vi "lighting control1.vi"() -> ()   [LabVIEW 2021]
uses:
  <vilib>/MakerHub/LINX/Public/Peripherals/Digital/Digital Write N Chans.vi
  9d78b206-77b7-4c78-aba5-ec40e68928b8.vi
  9e639ab3-c25c-4c4a-bd12-325d10f84e49.vi
  <vilib>/MakerHub/LINX/Private/Local IO/LinxDigitalWrite.vi
  <vilib>/MakerHub/LINX/Public/Utilities/Check Channel.vi
  <vilib>/MakerHub/LINX/Private/Local IO/LinxI2cWrite.vi
  <vilib>/MakerHub/LINX/Public/Utilities/Open Serial.vi
  <vilib>/Utility/file.llb/Write Delimited Spreadsheet (string).vi
  <vilib>/MakerHub/LINX/Private/Utilties/Generate Error.vi
  <vilib>/addons/Fuzzy Logic/FL Fuzzy Controller (MISO).vi
  <vilib>/Utility/file.llb/Write Delimited Spreadsheet (DBL).vi
  <vilib>/MakerHub/LINX/LMH-LINX.lvlib
  <vilib>/addons/Fuzzy Logic/NI_Fuzzy_Logic_API.lvlib
panel:
  out "no lamps":dbl
  out "fuzzy output":dbl
  out "no lamps":dbl
  out "fuzzy output":dbl
  out "indoor real":dbl
  in  "?":bool[](array[boolean])
  in  "?":bool[](array[boolean])
  in  "?":bool[](array[boolean])
  in  "Relay channels 3":dbl[](array[numeric])
  in  "outer stop":bool
  in  "inner stop":bool
  in  "channel name":string[](array[string])
  in  "Relay channels 2":dbl[](array[numeric])
  in  "Array 16":bool[](array[boolean])
  in  "Array 15":bool[](array[boolean])
  in  "?":bool[](array[boolean])
  in  "?":bool[](array[boolean])
  in  "?":bool[](array[boolean])
  in  "?":bool[](array[boolean])
  in  "?":bool[](array[boolean])
  in  "?":bool[](array[boolean])
  out "indoor from regr":dbl
  out "outdoor 2":dbl
  in  "Array 8":bool[](array[boolean])
  in  "Array 7":bool[](array[boolean])
  in  "?":bool[](array[boolean])
  in  "?":bool[](array[boolean])
  in  "?":bool[](array[boolean])
  in  "?":bool[](array[boolean])
  in  "?":bool[](array[boolean])
  in  "?":bool[](array[boolean])
  in  "Relay channels":dbl[](array[numeric])
  out "outdoor":dbl
  out "indoor":dbl
  # "CSV COLUMN CONFIG"
  # "RELAY ARDUINO CHANNELS"
  # "OFF CONFIG"
  # "DATA"
  # "BULB CASE CONFIG"
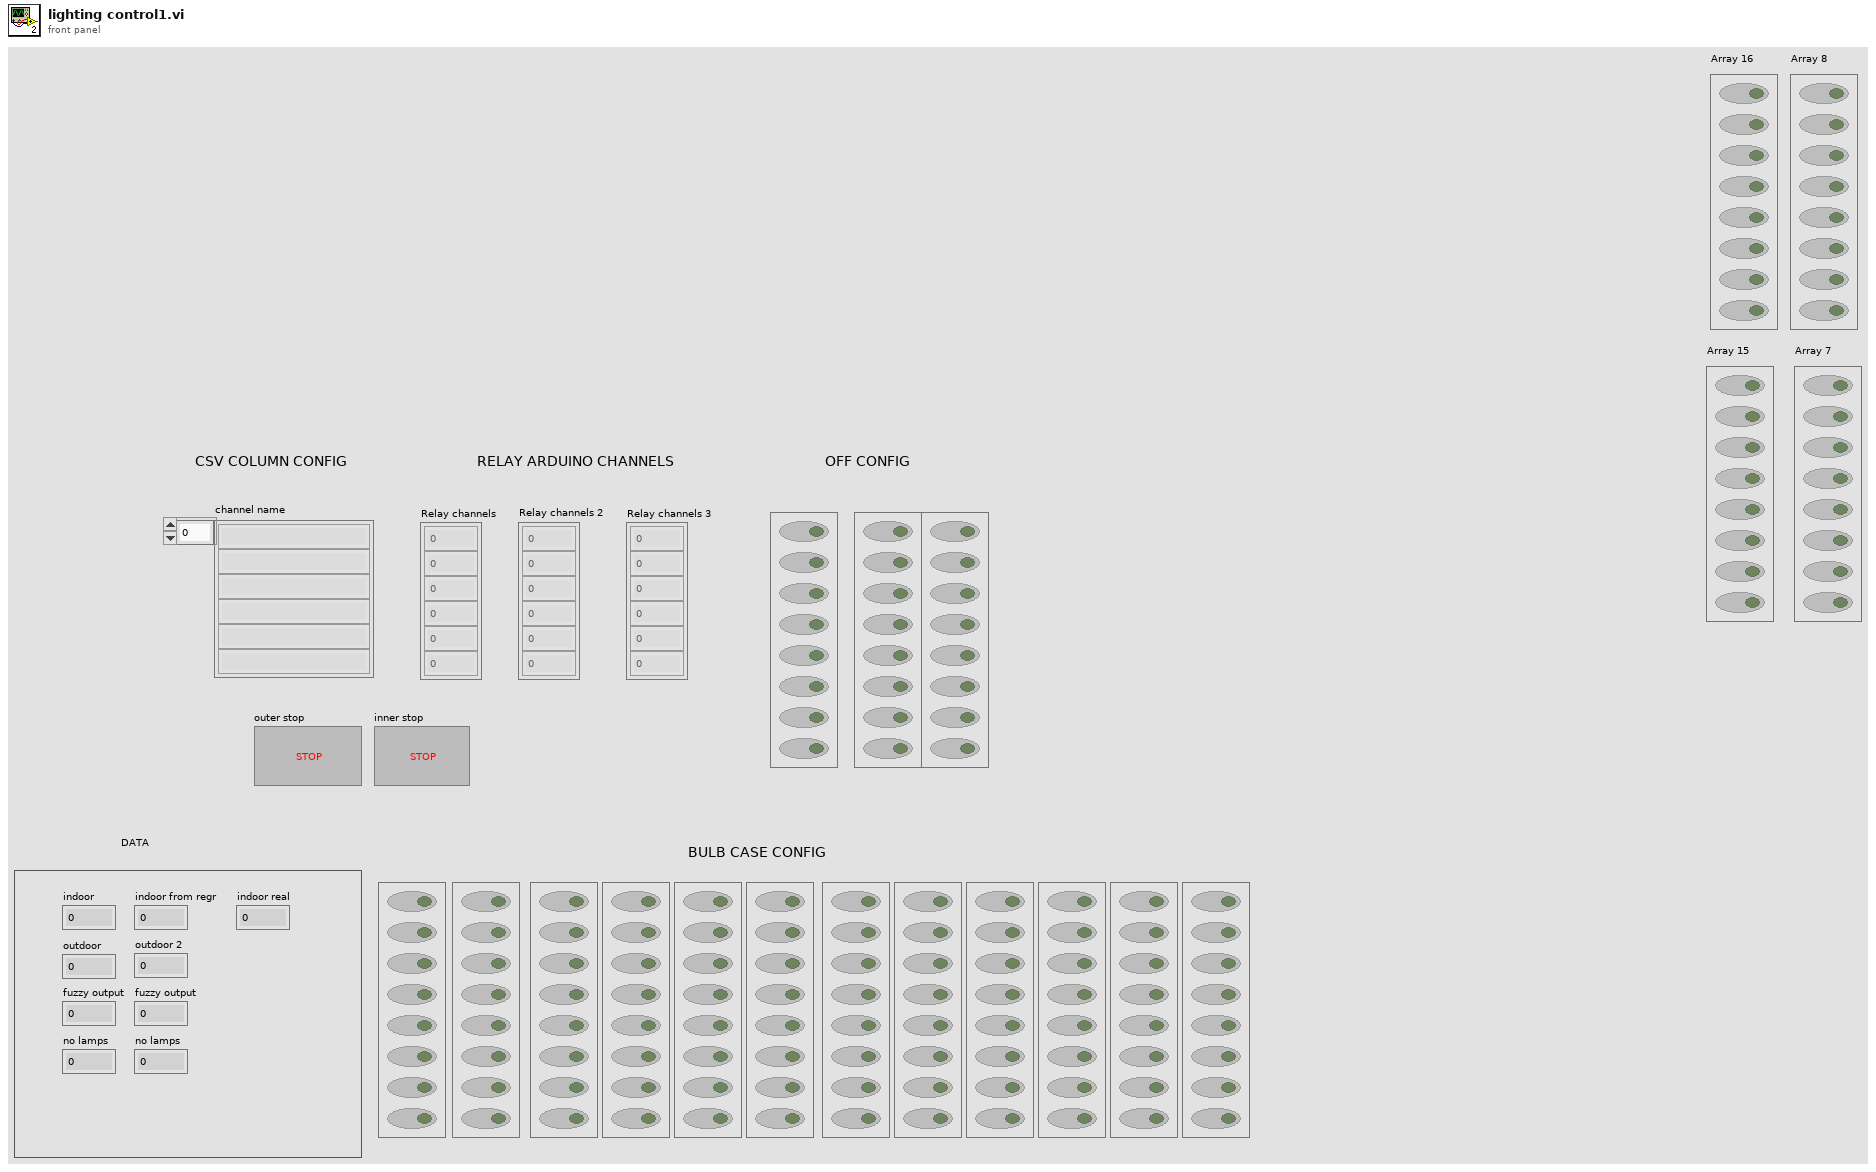
[diagram p1: front panel]
types:
  T1 = typedef "LMH-LINX.lvlib/LINX Ref.ctl" = cluster{"IO":T2, "Interface":T3, "LINX Device Config":T4}
  T2 = typedef "LMH-LINX.lvlib/Platform.ctl" = enum16{"Remote", "Local"}
  T3 = typedef "LMH-LINX.lvlib/Interface.ctl" = enum16{"Serial", "TCP"}
  T4 = typedef "LMH-LINX.lvlib/Device.lvlib/LINX Device Config.ctl" = cluster{"Interface":T3, "COM Port":refnum<visa-resource-name>, "TCP Configuration":T5, "Device Family":u8, "Device ID":u8, "Device Name":string, "TCP Ref":refnum<k5>, "Channels":T6}
  T5 = typedef "LMH-LINX.lvlib/Device.lvlib/TCP Config.ctl" = cluster{"IP Address":string, "Port":u16}
  T6 = typedef "LMH-LINX.lvlib/Channels.ctl" = cluster{"DI":u8[], "DO":u8[], "AI":u8[], "AO":u8[], "PWM":u8[], "QE":u8[], "UART":u8[], "I2C 2":u8[], "SPI":u8[], "CAN":u8[], "Servo":u8[], "AI Ref (V)":dbl, "AI Resolution (Bits)":u8, "AO Ref (V)":dbl, "AO Resolution (Bits)":u8}
  T7 = typedef "NI_Fuzzy_Logic_API.lvlib/FL System.ctl" = cluster{"input variables":T8[], "output variables":T8[], "rules":T11[], "defuzzification method":T17, "description":string, "user MF interpolating polynomials":T18[]}
  T8 = typedef "NI_Fuzzy_Logic_API.lvlib/FL Variable.ctl" = cluster{"name":string, "range":dbl[], "MFs":T9[]}
  T9 = typedef "NI_Fuzzy_Logic_API.lvlib/FL Membership Function.ctl" = cluster{"name":string, "shape":T10, "points":dbl[], "color":u32, "user-defined shape index":i32}
  T10 = typedef "NI_Fuzzy_Logic_API.lvlib/FL Membership Function Shape.ctl" = u16
  T11 = typedef "NI_Fuzzy_Logic_API.lvlib/FL Rule.ctl" = cluster{"antecedents":T12[], "antecedent connective":T14, "consequents":T15[], "consequent implication":T16, "degree of support":dbl}
  T12 = typedef "NI_Fuzzy_Logic_API.lvlib/FL Antecedent.ctl" = cluster{"Var Index":i32, "MF Index":i32, "Cond":T13}
  T13 = typedef "NI_Fuzzy_Logic_API.lvlib/FL Modifier.ctl" = u16
  T14 = typedef "NI_Fuzzy_Logic_API.lvlib/FL Antecedent Connective.ctl" = u16
  T15 = typedef "NI_Fuzzy_Logic_API.lvlib/FL Consequent.ctl" = cluster{"Var Index":i32, "MF Index":i32, "Cond":T13}
  T16 = typedef "NI_Fuzzy_Logic_API.lvlib/FL Consequent Implication.ctl" = u16
  T17 = typedef "NI_Fuzzy_Logic_API.lvlib/FL Defuzzification.ctl" = u16
  T18 = typedef "NI_Fuzzy_Logic_API.lvlib/FL Interpolating polynomials.ctl" = cluster{"X":dbl[], "Y":dbl[], "Y(x) coeff":dbl[][], "X(y) coeff":dbl[][], "Area(y) coeff":dbl[][], "coa_x(y) coeff":dbl[][]}
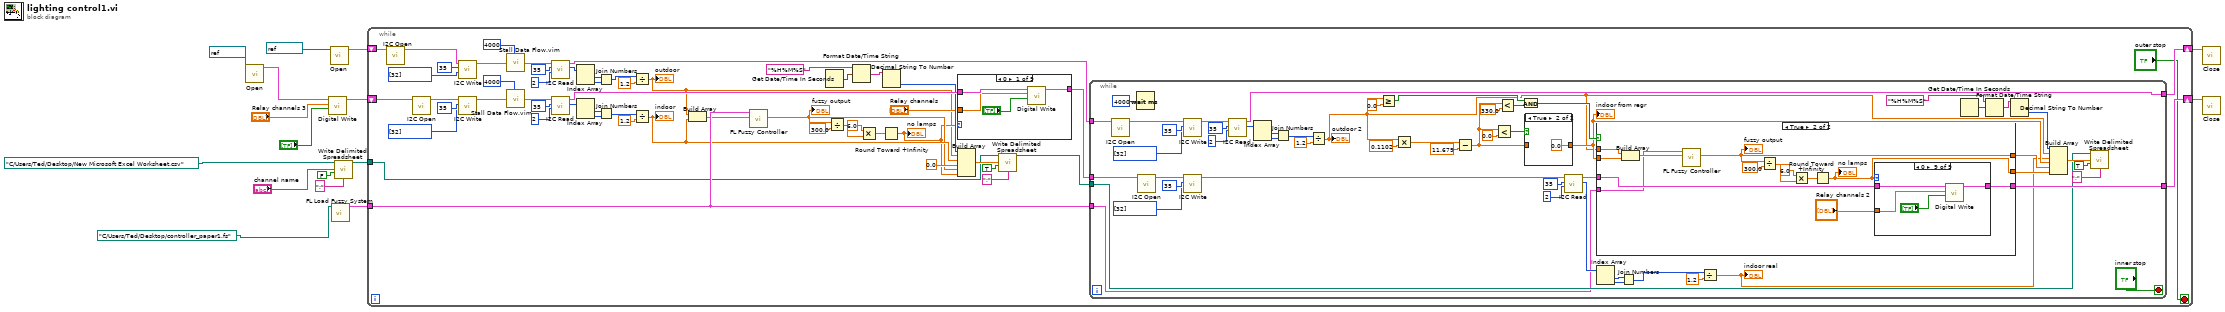
[diagram p0: block diagram]
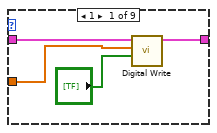
[diagram p4: hidden frame]
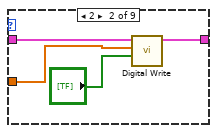
[diagram p5: hidden frame]
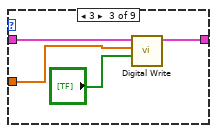
[diagram p6: hidden frame]
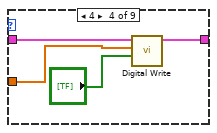
[diagram p7: hidden frame]
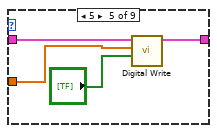
[diagram p8: hidden frame]
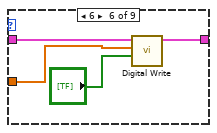
[diagram p9: hidden frame]
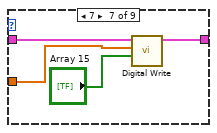
[diagram p10: hidden frame]
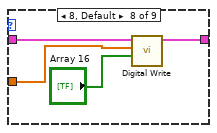
[diagram p11: hidden frame]
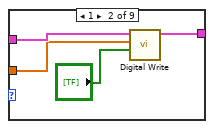
[diagram p12: hidden frame]
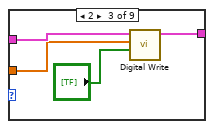
[diagram p13: hidden frame]
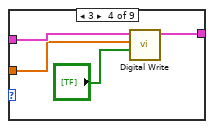
[diagram p14: hidden frame]
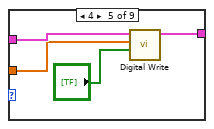
[diagram p15: hidden frame]
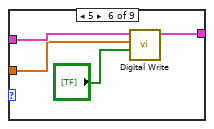
[diagram p16: hidden frame]
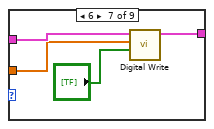
[diagram p17: hidden frame]
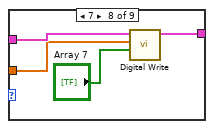
[diagram p18: hidden frame]
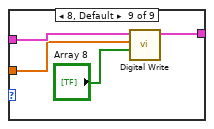
[diagram p19: hidden frame]
diagram:
  n1 = call-poly <vilib>:"Open.vi"("Serial Port"=refnum<visa-resource-name> "COM4") -> ("LINX Resource"=w2:T1)  [unwired: 8 in, 2 out]
  n2 = call-poly <vilib>:"Digital Write.vi"("Values"="?", "DO Channels"="Relay channels 3", "LINX Resource"=w2) -> ("LINX Resource"=w1:T1)  [unwired: 7 in, 1 out]
  n3 = call-poly <vilib>:"Open.vi"("Serial Port"=refnum<visa-resource-name> "COM5") -> ("LINX Resource"=w16:T1)  [unwired: 8 in, 2 out]
  n4 = call <vilib>:"FL Load Fuzzy System.vi"("file path"=path "C:/Users/Ted/Desktop/controller_paper1.fs") -> ("fuzzy system out"=w5:T7)  [unwired: 9 in, 1 out]
  n5 = call-poly <vilib>:"Write Delimited Spreadsheet.vi"("file path (dialog if empty)"=path "C:/Users/Ted/Desktop/New Microsoft Excel Worksheet.csv", "1D data"="channel name", "append to file? (new file:F)"=FALSE, "delimiter (\\t)"=";" ("delimiter (\\t)")) -> ("new file path (Not A Path if cancelled)"=w6:path)  [unwired: 10 in, 1 out]
  n6 = while {
    tunnel: w6 -> [w18]
    tunnel: w5 -> [w46]
    shift-right: [w48] -> w12
    shift-left: w1 -> [w61]
    shift-right: [w47] -> w11
    shift-left: w16 -> [w51]
    stop <- "outer stop" stop-if-true
    n7 = call <vilib>:"I2C Open.vi"("LINX Resource"=w51) -> ("LINX Resource"=w60:T1)  [unwired: 9 in, 1 out]
    n8 = call <vilib>:"I2C Open.vi"("LINX Resource"=w61) -> ("LINX Resource"=w71:T1)  [unwired: 9 in, 1 out]
    n9 = call <vilib>:"I2C Write.vi"("Data"=u8[] [32], "I2C Slave Address (0)"=u8 35, "LINX Resource"=w60) -> ("LINX Resource"=w41:T1)  [unwired: 7 in, 1 out]
    n10 = call <vilib>:"I2C Write.vi"("Data"=u8[] [32], "I2C Slave Address (0)"=u8 35, "LINX Resource"=w71) -> ("LINX Resource"=w44:T1)  [unwired: 7 in, 1 out]
    n11 = call "Stall Data Flow.vim"("value in"=w41, "milliseconds to wait"=u32 4000) -> ("value out"=w40:T1)  [unwired: 1 out]
    n12 = call "Stall Data Flow.vim"("value in"=w44, "milliseconds to wait"=u32 4000) -> ("value out"=w43:T1)  [unwired: 1 out]
    n13 = call <vilib>:"I2C Read.vi"("Bytes To Read"=u8 2, "I2C Slave Address (0)"=u8 35, "LINX Resource"=w40) -> ("Data"=w50:u8[], "LINX Resource"=w49:T1)  [unwired: 6 in, 1 out]
    n14 = call <vilib>:"I2C Read.vi"("Bytes To Read"=u8 2, "I2C Slave Address (0)"=u8 35, "LINX Resource"=w43) -> ("Data"=w68:u8[], "LINX Resource"=w45:T1)  [unwired: 6 in, 1 out]
    n15 = Index Array(array=w50) -> (element #1=w57:u8, element #2=w56:u8)  [unwired: 2 in]
    n16 = Index Array(array=w68) -> (element #1=w67:u8, element #2=w66:u8)  [unwired: 2 in]
    n17 = Join Numbers(hi=w57, lo=w56) -> ((hi.lo)=w54:u16)
    n18 = Join Numbers(hi=w67, lo=w66) -> ((hi.lo)=w64:u16)
    n19 = Divide(x=w54, y=1.2) -> (x/y=w17:dbl)
    "outdoor" <- w17
    n20 = Divide(x=w64, y=1.2) -> (x/y=w37:dbl)
    "indoor" <- w37
    n21 = Build Array(w17, w37) -> (w36:dbl[])
    n22 = call-poly <vilib>:"FL Fuzzy Controller.vi"("input values"=w36, "fuzzy system in"=w46) -> ("output value"=w20:dbl)  [unwired: 5 in, 4 out]
    "fuzzy output" <- w20
    n23 = Get Date/Time In Seconds() -> (seconds since 1Jan1904=w31:timestamp)
    n24 = Divide(x=w20, y=300.0) -> (x/y=w34:dbl)
    n25 = Format Date/Time String(time format string (%c)="%H%M%S", seconds (now)=w31) -> (date/time string=w29:string)  [unwired: 1 in]
    n26 = Multiply(x=6.0, y=w34) -> (x*y=w23:dbl)
    n27 = Decimal String To Number(string=w29) -> (number=w28:i32)  [unwired: 2 in, 1 out]
    n28 = Round Toward +Infinity(x=w23) -> (ceil(x): smallest int >= x=w19:dbl)
    "no lamps" <- w19
    n29 = case shown="0" w19 {
      tunnel: w45 -> [w181 w185 w188 w193 w196 w200 w205 w209 w213]
      tunnel: [w180 w184 w189 w192 w197 w201 w204 w208 w212] -> w32
      tunnel: "Relay channels" -> [w179 w182 w187 w191 w195 w199 w202 w207 w210]
      frame 0 {
        n30 = call-poly <vilib>:"Digital Write.vi"("Values"="?", "DO Channels"=w179, "LINX Resource"=w181) -> ("LINX Resource"=w180:T1)  [unwired: 7 in, 1 out]
      }
      frame 1 {
        n31 = call-poly <vilib>:"Digital Write.vi"("Values"="?", "DO Channels"=w182, "LINX Resource"=w185) -> ("LINX Resource"=w184:T1)  [unwired: 7 in, 1 out]
      }
      frame 2 {
        n32 = call-poly <vilib>:"Digital Write.vi"("Values"="?", "DO Channels"=w187, "LINX Resource"=w188) -> ("LINX Resource"=w189:T1)  [unwired: 7 in, 1 out]
      }
      frame 3 {
        n33 = call-poly <vilib>:"Digital Write.vi"("Values"="?", "DO Channels"=w191, "LINX Resource"=w193) -> ("LINX Resource"=w192:T1)  [unwired: 7 in, 1 out]
      }
      frame 4 {
        n34 = call-poly <vilib>:"Digital Write.vi"("Values"="?", "DO Channels"=w195, "LINX Resource"=w196) -> ("LINX Resource"=w197:T1)  [unwired: 7 in, 1 out]
      }
      frame 5 {
        n35 = call-poly <vilib>:"Digital Write.vi"("Values"="?", "DO Channels"=w199, "LINX Resource"=w200) -> ("LINX Resource"=w201:T1)  [unwired: 7 in, 1 out]
      }
      frame 6 {
        n36 = call-poly <vilib>:"Digital Write.vi"("Values"="?", "DO Channels"=w202, "LINX Resource"=w205) -> ("LINX Resource"=w204:T1)  [unwired: 7 in, 1 out]
      }
      frame 7 {
        n37 = call-poly <vilib>:"Digital Write.vi"("Values"="Array 7", "DO Channels"=w207, "LINX Resource"=w209) -> ("LINX Resource"=w208:T1)  [unwired: 7 in, 1 out]
      }
      frame 8, Default {
        n38 = call-poly <vilib>:"Digital Write.vi"("Values"="Array 8", "DO Channels"=w210, "LINX Resource"=w213) -> ("LINX Resource"=w212:T1)  [unwired: 7 in, 1 out]
      }
    }
    n39 = Build Array(w28, w17, w37, 0.0 ("element"), w20, w19) -> (w27:dbl[])
    n40 = call-poly <vilib>:"Write Delimited Spreadsheet.vi"("file path (dialog if empty)"=w18, "1D data"=w27, "append to file? (new file:F)"=TRUE, "delimiter (\\t)"=";" ("delimiter (\\t)")) -> ("new file path (Not A Path if cancelled)"=w25:path)  [unwired: 10 in, 1 out]
    n41 = while {
      tunnel: w32 -> [w103]
      tunnel: w49 -> [w102]
      tunnel: [w101] -> w48
      tunnel: [w100] -> w47
      tunnel: w25 -> [w93]
      tunnel: w46 -> [w90]
      stop <- "inner stop" stop-if-true
      n42 = call <vilib>:"I2C Open.vi"("LINX Resource"=w102) -> ("LINX Resource"=w125:T1)  [unwired: 9 in, 1 out]
      n43 = Wait (ms)(milliseconds to wait=u32 4000) -> ()  [unwired: 1 out]
      n44 = call <vilib>:"I2C Open.vi"("LINX Resource"=w103) -> ("LINX Resource"=w115:T1)  [unwired: 9 in, 1 out]
      n45 = call <vilib>:"I2C Write.vi"("Data"=u8[] [32], "I2C Slave Address (0)"=u8 35, "LINX Resource"=w125) -> ("LINX Resource"=w89:T1)  [unwired: 7 in, 1 out]
      n46 = call <vilib>:"I2C Write.vi"("Data"=u8[] [32], "I2C Slave Address (0)"=u8 35, "LINX Resource"=w115) -> ("LINX Resource"=w107:T1)  [unwired: 7 in, 1 out]
      n47 = call <vilib>:"I2C Read.vi"("Bytes To Read"=u8 2, "I2C Slave Address (0)"=u8 35, "LINX Resource"=w89) -> ("Data"=w116:u8[], "LINX Resource"=w100:T1)  [unwired: 6 in, 1 out]
      n48 = Index Array(array=w116) -> (element #1=w122:u8, element #2=w121:u8)  [unwired: 2 in]
      n49 = Join Numbers(hi=w122, lo=w121) -> ((hi.lo)=w119:u16)
      n50 = Divide(x=w119, y=1.2) -> (x/y=w73:dbl)
      "outdoor 2" <- w73
      n51 = Greater Or Equal?(x=w73, y=0.0) -> (x >= y?=w86:bool)
      n52 = Multiply(x=w73, y=0.1102) -> (x*y=w85:dbl)
      n53 = Subtract(x=w85, y=11.679) -> (x-y=w77:dbl)
      n54 = Less?(x=w77, y=0.0) -> (x < y?=w79:bool)
      n55 = Less?(x=w77, y=330.0) -> (x < y?=w87:bool)
      n56 = And(x=w86, y=w87) -> (x .and. y?=w80:bool)
      n57 = case shown="True" w79 {
        tunnel: [w126 0.0] -> w76
        tunnel: w77 -> [w126 _]
        frame False {
        }
        frame True {
        }
      }
      "indoor from regr" <- w76
      n58 = call <vilib>:"I2C Read.vi"("Bytes To Read"=u8 2, "I2C Slave Address (0)"=u8 35, "LINX Resource"=w107) -> ("Data"=w105:u8[], "LINX Resource"=w104:T1)  [unwired: 6 in, 1 out]
      n59 = case shown="True" w80 {
        tunnel: w73 -> [_ w130]
        tunnel: w104 -> [w128 w136]
        tunnel: [w128 w135] -> w101
        tunnel: [_ w134] -> w74
        tunnel: [_ w131] -> w75
        tunnel: w90 -> [_ w133]
        tunnel: w76 -> [_ w129]
        frame False {
        }
        frame True {
          n60 = Build Array(w130, w129) -> (w141:dbl[])
          n61 = call-poly <vilib>:"FL Fuzzy Controller.vi"("input values"=w141, "fuzzy system in"=w133) -> ("output value"=w134:dbl)  [unwired: 5 in, 4 out]
          "fuzzy output" <- w134
          n62 = Divide(x=w134, y=300.0) -> (x/y=w139:dbl)
          n63 = Multiply(x=6.0, y=w139) -> (x*y=w132:dbl)
          n64 = Round Toward +Infinity(x=w132) -> (ceil(x): smallest int >= x=w131:dbl)
          "no lamps" <- w131
          n65 = case shown="0" w131 {
            tunnel: w136 -> [w145 w148 w153 w156 w160 w165 w169 w173 w176]
            tunnel: [w144 w149 w152 w157 w161 w164 w168 w172 w175] -> w135
            tunnel: "Relay channels 2" -> [w142 w147 w151 w155 w159 w162 w167 w170 w174]
            frame 1 {
              n66 = call-poly <vilib>:"Digital Write.vi"("Values"="?", "DO Channels"=w142, "LINX Resource"=w145) -> ("LINX Resource"=w144:T1)  [unwired: 7 in, 1 out]
            }
            frame 2 {
              n67 = call-poly <vilib>:"Digital Write.vi"("Values"="?", "DO Channels"=w147, "LINX Resource"=w148) -> ("LINX Resource"=w149:T1)  [unwired: 7 in, 1 out]
            }
            frame 3 {
              n68 = call-poly <vilib>:"Digital Write.vi"("Values"="?", "DO Channels"=w151, "LINX Resource"=w153) -> ("LINX Resource"=w152:T1)  [unwired: 7 in, 1 out]
            }
            frame 4 {
              n69 = call-poly <vilib>:"Digital Write.vi"("Values"="?", "DO Channels"=w155, "LINX Resource"=w156) -> ("LINX Resource"=w157:T1)  [unwired: 7 in, 1 out]
            }
            frame 5 {
              n70 = call-poly <vilib>:"Digital Write.vi"("Values"="?", "DO Channels"=w159, "LINX Resource"=w160) -> ("LINX Resource"=w161:T1)  [unwired: 7 in, 1 out]
            }
            frame 6 {
              n71 = call-poly <vilib>:"Digital Write.vi"("Values"="?", "DO Channels"=w162, "LINX Resource"=w165) -> ("LINX Resource"=w164:T1)  [unwired: 7 in, 1 out]
            }
            frame 7 {
              n72 = call-poly <vilib>:"Digital Write.vi"("Values"="Array 15", "DO Channels"=w167, "LINX Resource"=w169) -> ("LINX Resource"=w168:T1)  [unwired: 7 in, 1 out]
            }
            frame 8, Default {
              n73 = call-poly <vilib>:"Digital Write.vi"("Values"="Array 16", "DO Channels"=w170, "LINX Resource"=w173) -> ("LINX Resource"=w172:T1)  [unwired: 7 in, 1 out]
            }
            frame 0 {
              n74 = call-poly <vilib>:"Digital Write.vi"("Values"="?", "DO Channels"=w174, "LINX Resource"=w176) -> ("LINX Resource"=w175:T1)  [unwired: 7 in, 1 out]
            }
          }
        }
      }
      n75 = Index Array(array=w105) -> (element #1=w112:u8, element #2=w111:u8)  [unwired: 2 in]
      n76 = Join Numbers(hi=w112, lo=w111) -> ((hi.lo)=w109:u16)
      n77 = Divide(x=w109, y=1.2) -> (x/y=w72:dbl)
      "indoor real" <- w72
      n78 = Get Date/Time In Seconds() -> (seconds since 1Jan1904=w99:timestamp)
      n79 = Format Date/Time String(time format string (%c)="%H%M%S", seconds (now)=w99) -> (date/time string=w97:string)  [unwired: 1 in]
      n80 = Decimal String To Number(string=w97) -> (number=w96:i32)  [unwired: 2 in, 1 out]
      n81 = Build Array(w96, w73, w72, w76, w74, w75) -> (w95:dbl[])
      n82 = call-poly <vilib>:"Write Delimited Spreadsheet.vi"("file path (dialog if empty)"=w93, "1D data"=w95, "append to file? (new file:F)"=TRUE, "delimiter (\\t)"=";" ("delimiter (\\t)")) -> ()  [unwired: 10 in, 2 out]
    }
  }
  n83 = call <vilib>:"Close.vi"("LINX Resource"=w11) -> ()  [unwired: 10 in, 1 out]
  n84 = call <vilib>:"Close.vi"("LINX Resource"=w12) -> ()  [unwired: 10 in, 1 out]
